vi "ProcessCurveData.vi"(11 "New Curve Values":T1) -> ()   [LabVIEW 2025]
uses:
  NewCurveDataEventArgs.ctl
  E:/PSCode/PalmSens_SDK/labview/PalmSens/Libraries/PalmSens.Core.Simplified.LabVIEW.dll
  Libraries/PalmSens.Core.Simplified.LabVIEW.dll
  LiveCurveResult.ctl
  MeasurementsResult.ctl
  MeasurementResults.ctl
  CurvesByMeasurement.ctl
  MeasurementInfo.ctl
  CurveInfo.ctl
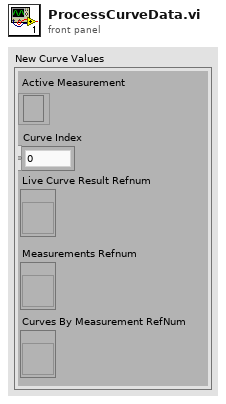
[diagram p1: front panel]
types:
  T1 = typedef "NewCurveDataEventArgs.ctl" = cluster{"Active Measurement":refnum<k24>, "Live Curve Result Refnum":refnum<vi>, "Measurements Refnum":refnum<vi>, "Curves By Measurement RefNum":refnum<vi>, "Curve Index":i32}
  T2 = typedef "CurvesByMeasurement.ctl" = map{refnum<k24>, T3}
  T3 = typedef "MeasurementInfo.ctl" = cluster{"Index":i32, "Is Measuring Refnum":refnum<vi>, "MeasurementEnded callback refnum":refnum<k27>, "SimpleCurveAdded callback refnum":refnum<k27>, "Live Curve Result Refnum":refnum<vi>, "Map":map{i32, T4}}
  T4 = typedef "CurveInfo.ctl" = cluster{"NewDataAdded callback refnum":refnum<k27>, "CurveFinished callback refnum":refnum<k27>}
  T5 = typedef "MeasurementsResult.ctl" = cluster{"Name":string, "Curves":T6, "Index":i32}[]
  T6 = typedef "MeasurementResults.ctl" = T7[]
  T7 = typedef "LiveCurveResult.ctl" = cluster{"X Label":string, "Y Label":string, "Name":string, "Index":i16, "Curve Values":cluster{"Values":cluster{"X Value":dbl, "Y Value":dbl}[], "Index":i16}}
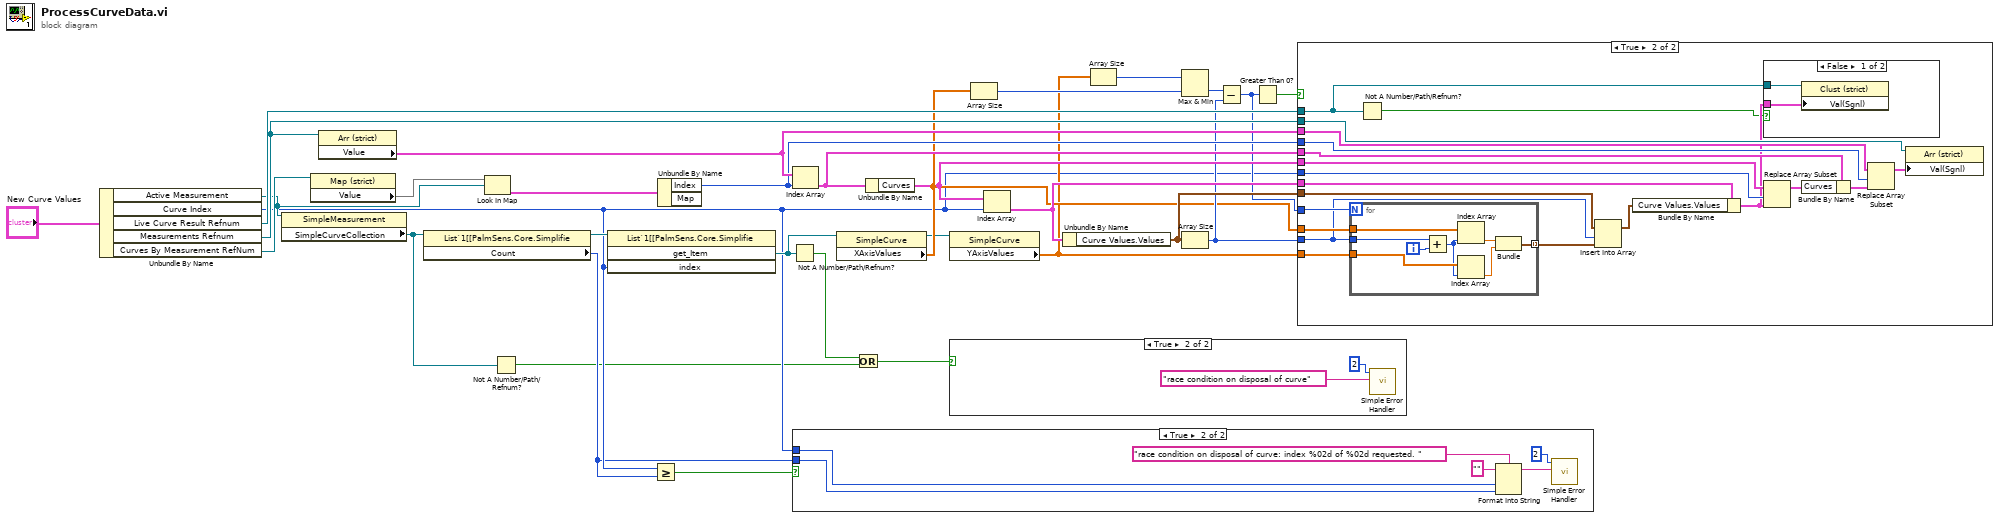
[diagram p0: block diagram]
diagram:
  n1 = Unbundle By Name("New Curve Values") -> ("Active Measurement"=w10:refnum<k24>, "Curve Index"=w6:i32, "Live Curve Result Refnum"=w27:refnum<vi>, "Measurements Refnum"=w31:refnum<vi>, "Curves By Measurement RefNum"=w15:refnum<vi>)
  n2 = property class="SimpleMeasurement"(reference=w10) -> ("SimpleCurveCollection"=w4:refnum<k24>)  [unwired: 1 in, 2 out]
  n3 = property class="Map (strict)"(reference=w15) -> ("Value"=w16:T2)  [unwired: 1 in, 2 out]
  n4 = property class="Arr (strict)"(reference=w31) -> ("Value"=w30:T5)  [unwired: 1 in, 2 out]
  n5 = property class="List`1[[PalmSens.Core.Simplifie"(reference=w4) -> (reference out=w9:refnum<k24>, "Count"=w5:i32)  [unwired: 1 in, 1 out]
  n6 = Look In Map(map=w16, key=w10) -> (value=w17:T3)  [unwired: 1 in, 1 out]
  n7 = Not A Number/Path/Refnum?(number/path/refnum=w4) -> (NaN/Path/Refnum?=w1:bool)
  n8 = invoke class="List`1[[PalmSens.Core.Simplifie" method="get_Item"(reference=w9, "index"=w6) -> ("get_Item"=w7:refnum<k24>)  [unwired: 2 in, 3 out]
  n9 = Greater Or Equal?(x=w6, y=w5) -> (x >= y?=w8:bool)
  n10 = Unbundle By Name(w17) -> ("Index"=w29:i32)  [unwired: 1 out]
  n11 = Not A Number/Path/Refnum?(number/path/refnum=w7) -> (NaN/Path/Refnum?=w3:bool)
  n12 = Index Array(array=w30, index=w29) -> (element=w28:cluster{"Name":string, "Curves":T6, "Index":i32})
  n13 = case shown="True" w8 {
    tunnel: w6 -> [_ w35]
    tunnel: w5 -> [_ w34]
    frame False {
    }
    frame True {
      n14 = Format Into String(format string="race condition on disposal of curve: index %02d of %02d requested. " ("error source (\" \")"), initial string="", w35, w34) -> (resulting string=w33:string)  [unwired: 1 in, 1 out]
      n15 = call <vilib>:"Simple Error Handler.vi"("error code (no error:0)"=2, "error source (\" \")"=w33) -> ()  [unwired: 3 in, 5 out]
    }
  }
  n16 = property class="SimpleCurve"(reference=w7) -> (reference out=w11:refnum<k24>, "XAxisValues"=w18:dbl[])  [unwired: 1 in, 1 out]
  n17 = Or(x=w3, y=w1) -> (x .or. y?=w2:bool)
  n18 = Unbundle By Name(w28) -> ("Curves"=w26:T6)
  n19 = property class="SimpleCurve"(reference=w11) -> ("YAxisValues"=w13:dbl[])  [unwired: 1 in, 2 out]
  n20 = case shown="True" w2 {
    frame False {
    }
    frame True {
      n21 = call <vilib>:"Simple Error Handler.vi"("error code (no error:0)"=2, "error source (\" \")"="race condition on disposal of curve" ("error source (\" \")")) -> ()  [unwired: 3 in, 5 out]
    }
  }
  n22 = Array Size(array=w18) -> (size(s)=w19:i32)
  n23 = Index Array(array=w26, index=w6) -> (element=w25:T7)
  n24 = Unbundle By Name(w25) -> ("Curve Values.Values"=w24:cluster{"X Value":dbl, "Y Value":dbl}[])
  n25 = Array Size(array=w13) -> (size(s)=w12:i32)
  n26 = Max & Min(x=w12, y=w19) -> (min(x,y)=w20:i32)  [unwired: 1 out]
  n27 = Array Size(array=w24) -> (size(s)=w23:i32)
  n28 = Subtract(x=w20, y=w23) -> (x-y=w22:i32)
  n29 = Greater Than 0?(x=w22) -> (x > 0?=w21:bool)
  n30 = case shown="True" w21 {
    tunnel: w18 -> [_ w59]
    tunnel: w13 -> [_ w58]
    tunnel: w22 -> [_ w57]
    tunnel: w23 -> [_ w55]
    tunnel: w24 -> [_ w56]
    tunnel: w25 -> [_ w52]
    tunnel: w26 -> [_ w51]
    tunnel: w6 -> [_ w50]
    tunnel: w27 -> [_ w40]
    tunnel: w28 -> [_ w49]
    tunnel: w29 -> [_ w46]
    tunnel: w30 -> [_ w45]
    tunnel: w31 -> [_ w43]
    frame False {
    }
    frame True {
      n31 = for {
        N: w57 -> [_]
        tunnel: w59 -> [w69]
        tunnel: w58 -> [w66]
        tunnel: [w63] -> w54 mode=indexing
        tunnel: w55 -> [w62]
        i -> [w68]
        n32 = Add(x=w62, y=w68) -> (x+y=w65:i32)
        n33 = Index Array(array=w69, index=w65) -> (element=w67:dbl)
        n34 = Index Array(array=w66, index=w65) -> (element=w64:dbl)
        n35 = Bundle(w67, w64) -> (w63:cluster{dbl, dbl})  [unwired: 1 in]
      }
      n36 = Not A Number/Path/Refnum?(number/path/refnum=w40) -> (NaN/Path/Refnum?=w41:bool)
      n37 = Insert Into Array(array=w56, index=w55, new element=w54) -> (w53:cluster{"X Value":dbl, "Y Value":dbl}[])
      n38 = Bundle By Name(cluster=w52, "Curve Values.Values"=w53) -> (w42:T7)
      n39 = case shown="False" w41 {
        tunnel: w40 -> [w61 _]
        tunnel: w42 -> [w60 _]
        frame False {
          n40 = property class="Clust (strict)"(reference=w61, "Val(Sgnl)"=w60) -> ()  [unwired: 1 in, 2 out]
        }
        frame True {
        }
      }
      n41 = Replace Array Subset(array=w51, new element=w42, index=w50) -> (w48:T6)
      n42 = Bundle By Name(cluster=w49, "Curves"=w48) -> (w47:cluster{"Name":string, "Curves":T6, "Index":i32})
      n43 = Replace Array Subset(array=w45, new element=w47, index=w46) -> (w44:T5)
      n44 = property class="Arr (strict)"(reference=w43, "Val(Sgnl)"=w44) -> ()  [unwired: 1 in, 2 out]
    }
  }
